vi "DVS_LabVIEW Controller.vi"() -> ()   [LabVIEW 2013]
doc: "This example demonstrates temperature control and monitoring.\n\nNote:\nBefore start this VI is it necessary:\n\n- preconfigure some specific parameters that are not supported by this driver (e.g. PV-I/O Type, Linearization type, Alarm Input Values... ) by Quick Codes, or by Eurotherm iTools or by instrument front panel controls\n- enter correct VISA Resource Descriptor, Device Address and Baud Rate into front-panel controls"
uses:
  <vilib>/Instr/_visa.llb/VISA Event Mechanism.ctl
  <vilib>/Instr/_visa.llb/Select Event Type.ctl
  <vilib>/Utility/file.llb/Write To Spreadsheet File (string).vi
  <vilib>/Instr/_visa.llb/VISA Configure Serial Port (Instr).vi
  <instrlib>/Keithley 24XX/Public/Data/Read (Single Point).vi
  <instrlib>/Keithley 24XX/Keithley 24XX.lvlib
panel:
  in  "stop":bool
  in  "Tab Control":T1(tab)
  in  "Add comments to the data file here and click anywhere outside\nthe comment box to save. The time at which the comment is\nsaved is recorded in the data file.":string
  in  "O2 PUMP":bool
  in  "QCM":bool
  out "Program Errors":errorcluster
  out "Starting Date/Time":string
  in  "Keithley 4200":bool
  in  "Keithley 2420":bool
  in  "J-KEM":bool
  in  "Automatically stop\nmeasurement?":bool
  in  "Stop after elapsed minutes":dbl
  out "Time Elapsed (min)":dbl caption="Elapsed Time (s)"
  in  "RapidOX":bool
  out "Frequency (Hz)":dbl format="%.6e"
  out "Resistance (Ohm)":dbl format="%.6e"
  out "Waveform Chart 7":T2(graph)
  out "Waveform Chart 5":cluster{dbl, dbl}(graph)
  out "Current Temp (C)":dbl
  in  "Temp Setpoint (C)":dbl=25.0
  out "Current Setpoint (C)":dbl
  out "Waveform Chart":cluster{dbl}(graph)
  out "Torr":dbl
  out "%":dbl
  out "atm":dbl
  in  "Com Port":i32(ring) items=["Com 1", "Com 2", "Com 3", "Com 4", "Com 5", "Com 6", "COM 7", "COM 8", "COM 9", "COM 10", "COM 11", "COM 12", "com 13", "COM 14"]
  in  "Baud Rate 2":i32(ring)=2 items=["2400", "4800", "9600", "19200", "38400", "57600", "115200"]
  in  "Com Port 2":i32(ring) items=["Com 1", "Com 2", "Com 3", "Com 4", "Com 5", "Com 6", "COM 7", "COM 8", "COM 9", "COM 10", "COM 11", "COM 12", "com 13", "COM 14"]
  out "Waveform Chart 6":cluster{dbl}(graph)
  out "O2 Concentration (PPM)":dbl
  out "Waveform Chart 4":cluster{"Resistance":sgl}(graph)
  out "Resistance (Ohm)":sgl
  in  "Measurement":enum16{"Resistor/Diode", "Transistor"}(ring)
  out "Waveform Chart 3":cluster{dbl}(graph)
  out "XY Graph":cluster{dbl[], dbl[]}(graph)
  out "Current (A)    Voltage (V)":dbl[][](array[numeric]) caption="appended array"
  out "Resistance (Ohm)":dbl
  # "Configuring Instrument\n \nPlease Wait......\n\nChart will update in 20 sec"
  # "Instruments Connected"
  # "COMMENT BOX"
  # "Instructions:\nSelect the instruments above which are connected, turned on, and configured to record data.\nRun the Pirani Control software, and make sure Pirani is saving a log of the temp/pressure/gas flow data. \nClick the RUN arrow on the LabVIEW toolbar, and wait for instruments to begin recording.\nTo end, click the red STOP button ONLY for instruments that are running.\nDO NOT press the STOP button on the toolbar."
  # "O2 Partial\nPressure"
  # "4-Point Resistance Measurement:\nSMU1 = Current Source, Voltmeter\nSMU2 = COM & GND"
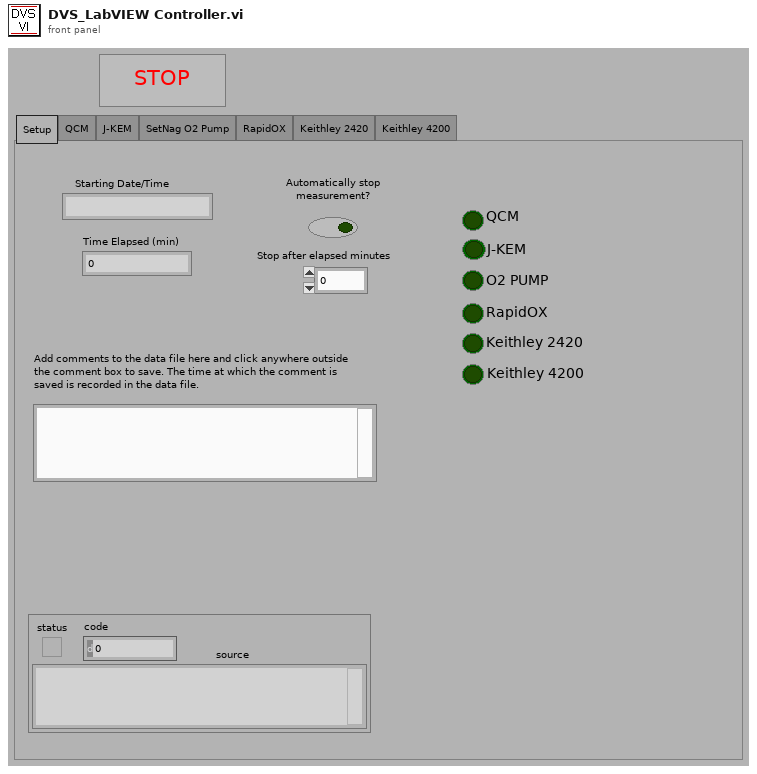
[diagram p1: front panel]
types:
  T1 = enum32{"Setup", "QCM", "J-KEM", "SetNag O2 Pump", "RapidOX", "Keithley 2420", "Keithley 4200"}
  T2 = cluster{"Frequency out":dbl, "Resistance out":dbl}
  T3 = enum16{"open", "open or create", "create or replace", "create", "open (read only)"}
  T4 = enum16{"no parity", "odd parity", "even parity", "mark parity", "space parity"}
  T5 = typedef "Select Event Type.ctl" = u32
  T6 = typedef "VISA Event Mechanism.ctl" = u16
  T7 = cluster{bool, "VISA resource name":refnum<visa-resource-name>, "error out":errorcluster}
  T8 = cluster{bool, "VISA resource name out":refnum<visa-resource-name>, "error out":errorcluster}
  T9 = cluster{bool, "VISA out":refnum<visa-resource-name>, "error out":errorcluster}
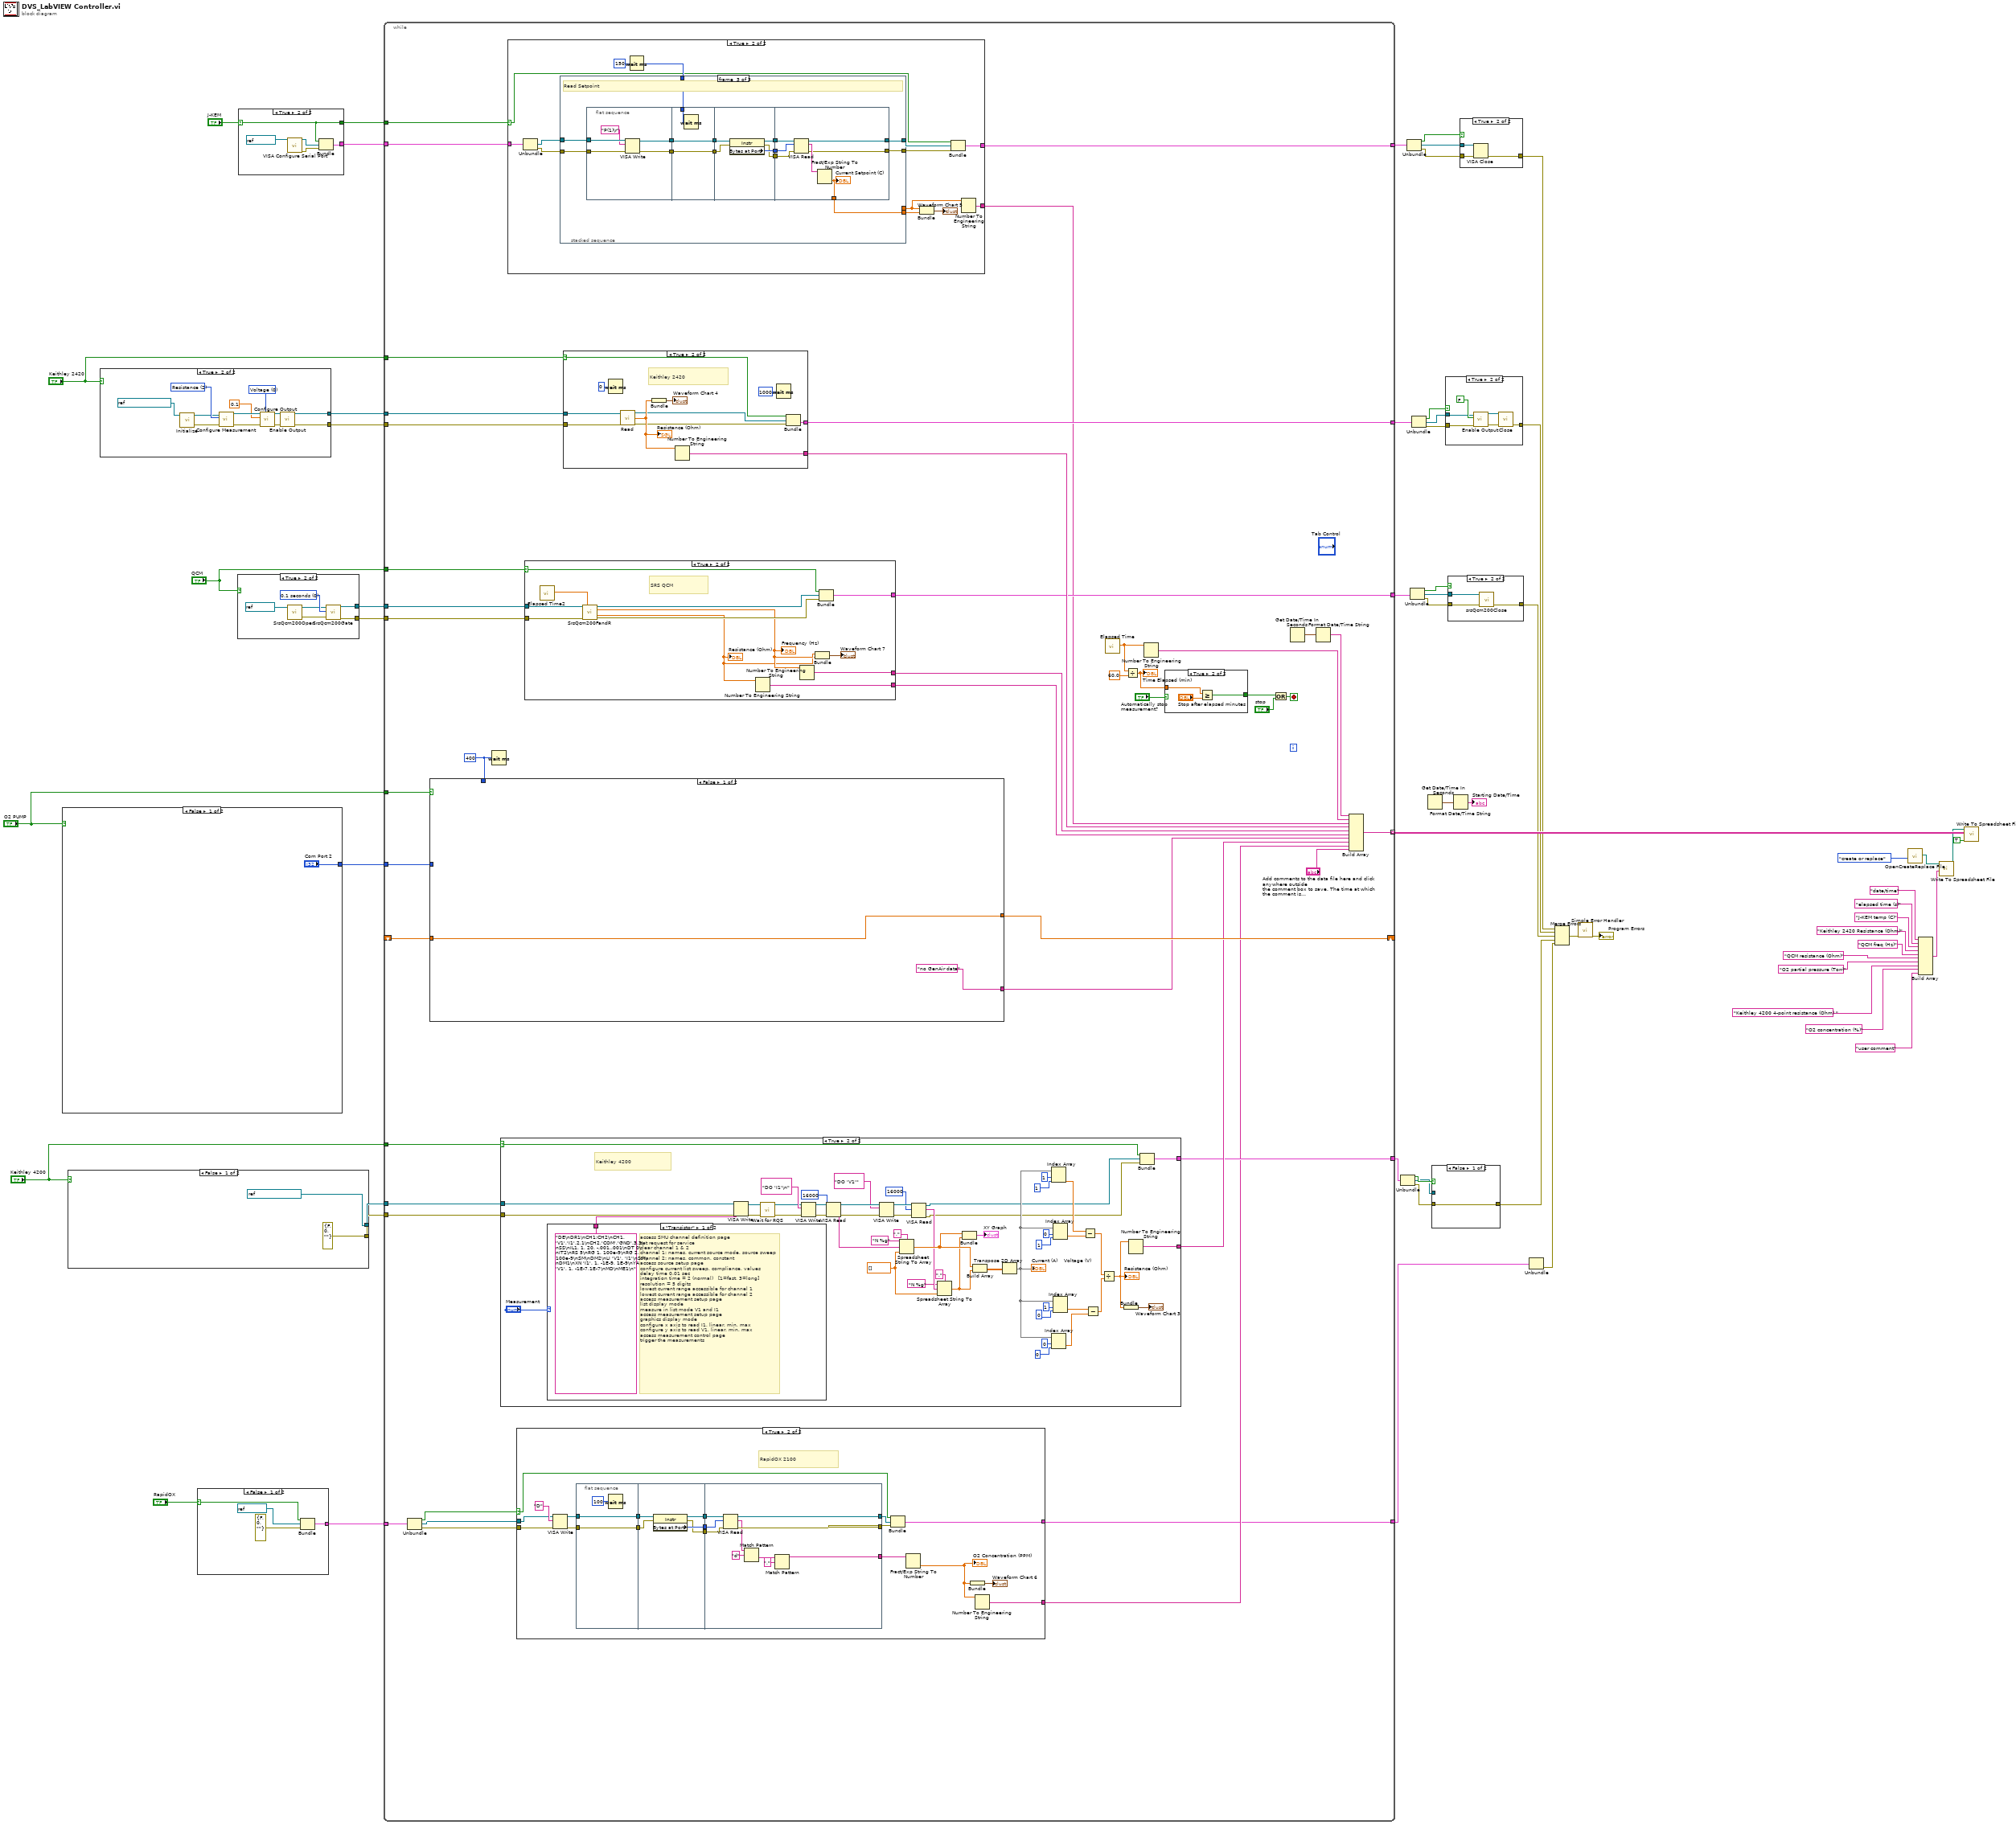
[diagram p0: block diagram]
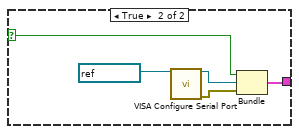
[diagram p2: hidden frame]
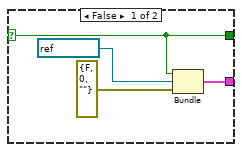
[diagram p4: hidden frame]
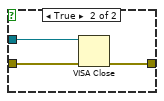
[diagram p5: hidden frame]
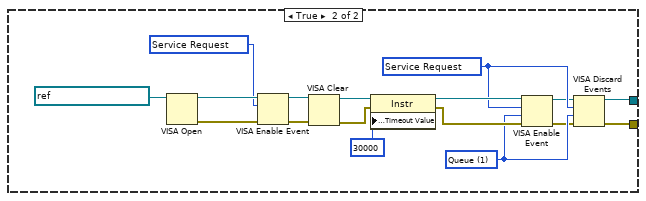
[diagram p6: hidden frame]
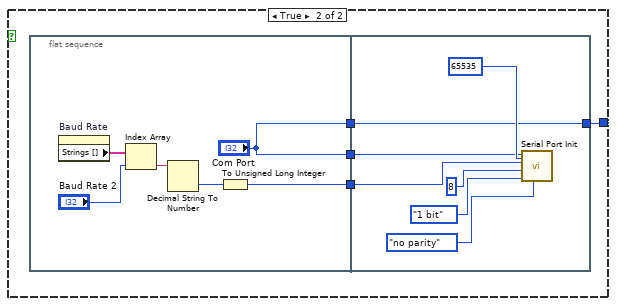
[diagram p7: hidden frame]
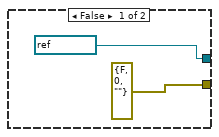
[diagram p9: hidden frame]
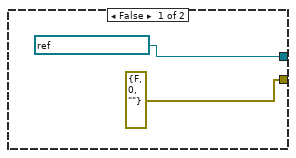
[diagram p11: hidden frame]
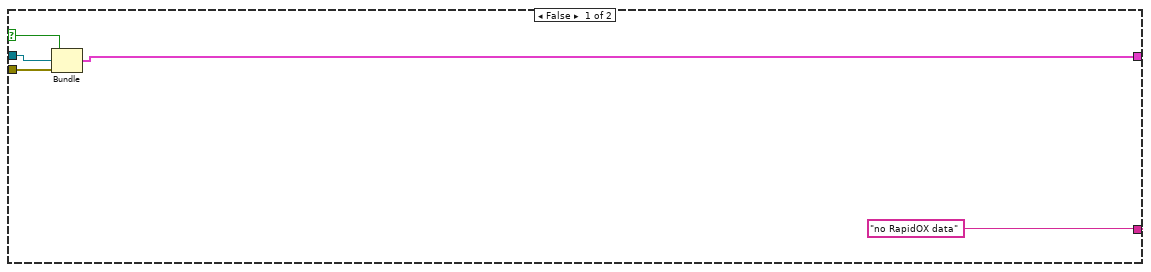
[diagram p12: hidden frame]
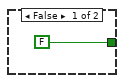
[diagram p13: hidden frame]
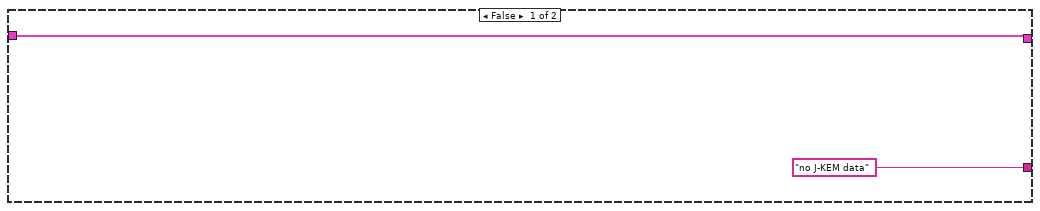
[diagram p14: hidden frame]
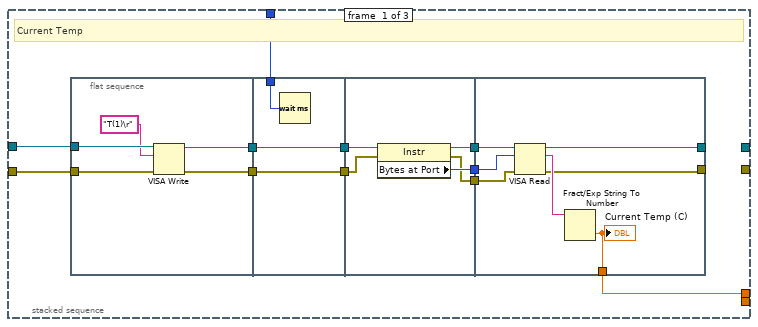
[diagram p15: hidden frame]
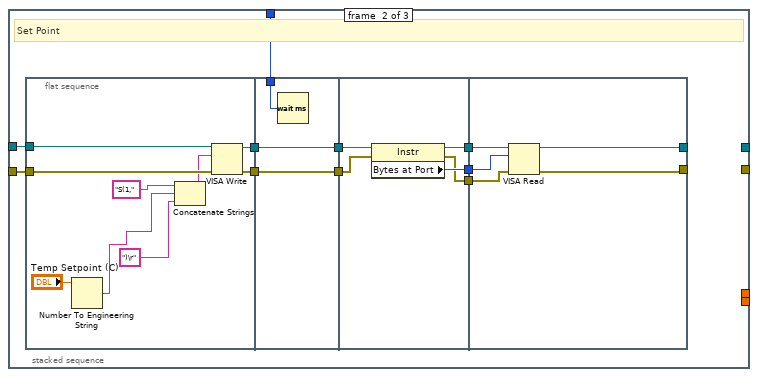
[diagram p16: hidden frame]
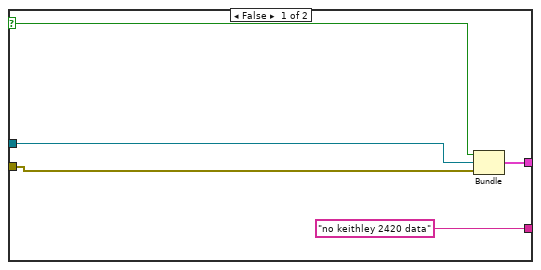
[diagram p17: hidden frame]
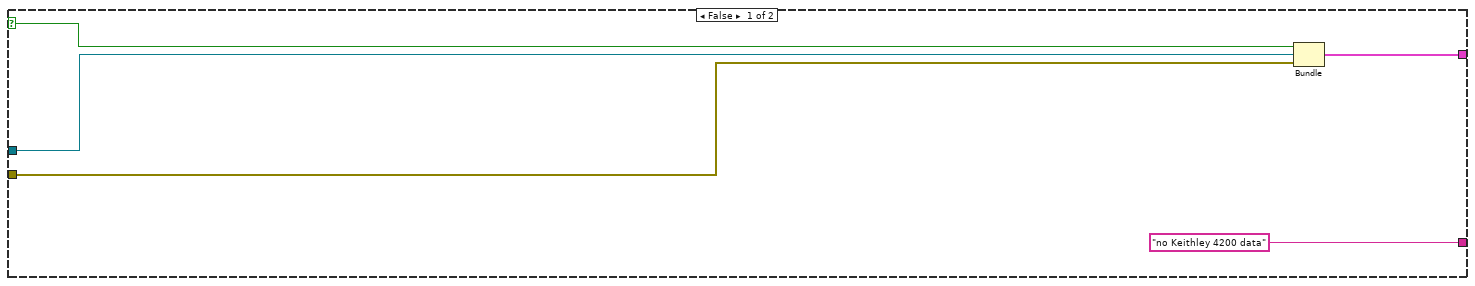
[diagram p18: hidden frame]
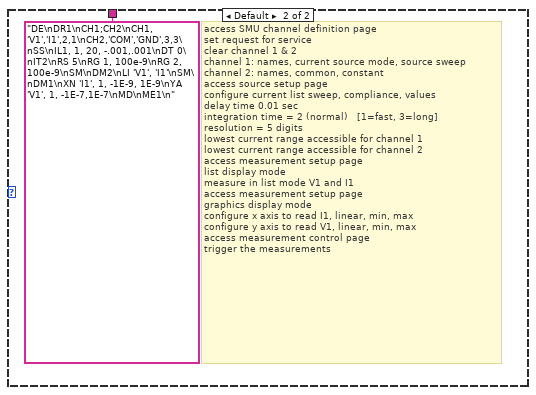
[diagram p19: hidden frame]
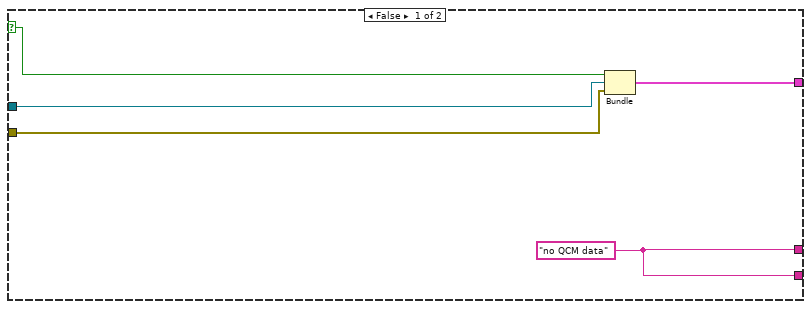
[diagram p20: hidden frame]
diagram:
  n1 = case shown="False" "O2 PUMP" {
    tunnel: ["Com Port 2" w60] -> w46
    frame False {
    }
    frame True {
      n2 = flat-sequence {
        tunnel: ["Com Port"] -> w63
        tunnel: [w65] -> w62
        tunnel: ["Com Port"] -> w61
        tunnel: w63 -> [w71]
        tunnel: w62 -> [w70]
        tunnel: w61 -> [w72]
        tunnel: [w72] -> w60
        frame #0 {
          n3 = property on="Baud Rate" class="Ring (strict)"() -> ("Strings []"=w67:string[])  [unwired: 2 in, 2 out]
          n4 = Index Array(array=w67, index="Baud Rate 2") -> (element=w68:string)
          n5 = Decimal String To Number(string=w68) -> (number=w66:i32)  [unwired: 2 in, 1 out]
          n6 = To Unsigned Long Integer(number=w66) -> (unsigned 32bit integer=w65:u32)
        }
        frame #1 {
          n7 = call <vilib>:"Serial Port Init.vi"("parity"=T4."no parity", "buffer size"=u16 65535, "stop bits"=enum16{"1 bit", "1.5 bits", "2 bits"}."1 bit", "data bits"=u16 8, "baud rate"=w70, "port number"=w71) -> ()  [unwired: 1 in, 1 out]
        }
      }
    }
  }
  n8 = case shown="False" "Keithley 4200" {
    tunnel: [refnum<visa-resource-name> "GPIB0::17::INSTR" ("VISA resource name") w80] -> w42
    tunnel: [errorcluster {"status"=FALSE, "code"=0, "source"=""} ("error out") w79] -> w41
    frame False {
    }
    frame True {
      w92 = T5 1073684491 items=["Service Request"=1073684491, "Trigger"=3221168138, "Clear"=1073684493, "VXI Signal"=1073684512, "VXI/VME Interrupt"=3221168161, "VXI/VME Sysfail"=1073684509, "VXI/VME Sysreset"=1073684510, "GPIB CIC"=1073684498, "GPIB Talk"=1073684499, "GPIB Listen"=1073684500, "PXI Interrupt"=1073684514, "Serial Break"=1073684515, "Serial TermChar"=1073684516, "Serial CTS"=1073684521, "Serial DSR"=1073684522, "Serial DCD"=1073684524, "Serial RI"=1073684526, "Serial Character"=1073684533, "USB Interrupt"=1073684535, "All Enabled"=1073709055] ("Event Type")
      w85 = T6 1 items=["Queue"=1] ("Mechanism Type")
      w84 = T5 1073684491 items=["Service Request"=1073684491, "Trigger"=3221168138, "Clear"=1073684493, "VXI Signal"=1073684512, "VXI/VME Interrupt"=3221168161, "VXI/VME Sysfail"=1073684509, "VXI/VME Sysreset"=1073684510, "GPIB CIC"=1073684498, "GPIB Talk"=1073684499, "GPIB Listen"=1073684500, "PXI Interrupt"=1073684514, "Serial Break"=1073684515, "Serial TermChar"=1073684516, "Serial CTS"=1073684521, "Serial DSR"=1073684522, "Serial DCD"=1073684524, "Serial RI"=1073684526, "Serial Character"=1073684533, "USB Interrupt"=1073684535, "All Enabled"=1073709055] ("Event Type")
      n9 = VISA Open(VISA resource name=refnum<visa-resource-name> "GPIB0::17::INSTR") -> (VISA resource name=w94:refnum<visa-resource-name>, error out=w95:errorcluster)  [unwired: 1 in, 3 out]
      n10 = VISA Enable Event(8:w95, 10:w92, 11:w94) -> (0:w91:errorcluster, 3:w90:refnum<visa-resource-name>)  [unwired: 1 out]
      n11 = VISA Clear(VISA resource name=w90, error in (no error)=w91) -> (VISA resource name out=w86:refnum<visa-resource-name>, error out=w87:errorcluster)
      n12 = property class="Instr"(reference=w86, error in=w87, "General Settings:Timeout Value"=u32 30000) -> (reference out=w88:refnum<visa-resource-name>, error out=w89:errorcluster)
      n13 = VISA Enable Event(8:w89, 9:w85, 10:w84, 11:w88) -> (0:w83:errorcluster, 3:w82:refnum<visa-resource-name>)
      n14 = VISA Discard Events(8:w83, 9:w85, 10:w84, 11:w82) -> (0:w79:errorcluster, 3:w80:refnum<visa-resource-name>)
    }
  }
  n15 = case shown="True" "Keithley 2420" {
    tunnel: [refnum<visa-resource-name> "GPIB1::24::INSTR" ("VISA resource name") w99] -> w52
    tunnel: [errorcluster {"status"=FALSE, "code"=0, "source"=""} ("error out") w98] -> w51
    frame False {
    }
    frame True {
      w103 = u16 0 items=["Voltage", "Current"] ("Source Mode  (0: Voltage)")
      w108 = u16 2 items=["Volts", "Current", "Resistance"] ("Function (0: Volts)")
      n16 = call <instrlib>:"Initialize.vi"("VISA resource name"=refnum<visa-resource-name> "GPIB1::24::INSTR") -> ("error out"=w100:errorcluster, "VISA resource name out"=w101:refnum<visa-resource-name>)  [unwired: 9 in]
      n17 = call <instrlib>:"Configure Measurement.vi"("error in (no error)"=w100, "Function (0: Volts)"=w108, "VISA resource name"=w101) -> ("error out"=w107:errorcluster, "VISA resource name out"=w106:refnum<visa-resource-name>)  [unwired: 7 in]
      n18 = call <instrlib>:"Configure Output.vi"("Source Mode  (0: Voltage)"=w103, "error in (no error)"=w107, "Output Level (0)"=0.1, "VISA resource name"=w106) -> ("error out"=w105:errorcluster, "VISA resource name out"=w104:refnum<visa-resource-name>)  [unwired: 6 in]
      n19 = call <instrlib>:"Enable Output.vi"("error in (no error)"=w105, "VISA resource name"=w104) -> ("error out"=w98:errorcluster, "VISA resource name out"=w99:refnum<visa-resource-name>)  [unwired: 8 in]
    }
  }
  n20 = case shown="False" "RapidOX" {
    selector: "RapidOX" -> [w110 w114]
    tunnel: [w111 w115] -> w4
    frame False {
      n21 = Bundle(w110, "VISA resource name"=refnum<visa-resource-name> "COM7", "error out"=errorcluster {"status"=FALSE, "code"=0, "source"=""}) -> (w111:T7)  [unwired: 1 in]
    }
    frame True {
      n22 = call-poly "VISA Configure Serial Port"("VISA resource name"=refnum<visa-resource-name> "COM7") -> ("VISA resource name out"=w117:refnum<visa-resource-name>, "error out"=w116:errorcluster)  [unwired: 13 in]
      n23 = Bundle(w114, "VISA resource name out"=w117, "error out"=w116) -> (w115:T8)  [unwired: 1 in]
    }
  }
  n24 = case shown="True" "QCM" {
    tunnel: [refnum<visa-resource-name> "COM6" ("VISA in") w122] -> w50
    tunnel: [errorcluster {"status"=FALSE, "code"=0, "source"=""} ("error out") w121] -> w49
    frame False {
    }
    frame True {
      w126 = u16 0 items=["0.1 seconds", "1.0 seconds", "10.0 seconds"] ("Gate in")
      n25 = call <instrlib>:"SrsQcm200Open.vi"("VISA in"=refnum<visa-resource-name> "COM6") -> ("error out"=w123:errorcluster, "VISA out"=w124:refnum<visa-resource-name>)  [unwired: 4 in]
      n26 = call <instrlib>:"SrsQcm200Gate.vi"("VISA in"=w124, "Gate in"=w126, "error in (no error)"=w123) -> ("VISA out"=w122:refnum<visa-resource-name>, "error out"=w121:errorcluster)  [unwired: 14 in, 1 out]
    }
  }
  n27 = case shown="True" "J-KEM" {
    selector: "J-KEM" -> [w127 w131]
    tunnel: [w128 w132] -> w28
    tunnel: [w127 w131] -> w20
    frame False {
      n28 = Bundle(w127, "VISA resource name"=refnum<visa-resource-name> "COM3", "error out"=errorcluster {"status"=FALSE, "code"=0, "source"=""}) -> (w128:T7)  [unwired: 1 in]
    }
    frame True {
      n29 = call-poly "VISA Configure Serial Port"("VISA resource name"=refnum<visa-resource-name> "COM3") -> ("VISA resource name out"=w134:refnum<visa-resource-name>, "error out"=w133:errorcluster)  [unwired: 13 in]
      n30 = Bundle(w131, "VISA resource name out"=w134, "error out"=w133) -> (w132:T8)  [unwired: 1 in]
    }
  }
  n31 = while {
    shift-right: [w177] -> _
    shift-left: _ -> [w176]
    tunnel: [w173] -> w54 mode=indexing
    tunnel: "Keithley 2420" -> [w169]
    tunnel: w52 -> [w171]
    tunnel: w51 -> [w170]
    tunnel: w50 -> [w168]
    tunnel: w49 -> [w167]
    tunnel: "QCM" -> [w165]
    tunnel: "O2 PUMP" -> [w154]
    tunnel: w46 -> [w164]
    tunnel: "Keithley 4200" -> [w158]
    tunnel: w42 -> [w163]
    tunnel: w41 -> [w162]
    tunnel: [w156] -> w40
    tunnel: [w155] -> w36
    tunnel: [w153] -> w32
    tunnel: w28 -> [w152]
    tunnel: [w151] -> w26
    tunnel: w20 -> [w149]
    tunnel: w4 -> [w141]
    tunnel: [w136] -> w2
    stop <- w147 stop-if-true
    w175 = u32 400 ("milliseconds to wait")
    n32 = Unbundle(w141) -> (w140:bool, "VISA resource name out"=w139:refnum<visa-resource-name>, "error out"=w138:errorcluster)
    n33 = case shown="False" w154 {
      tunnel: [w427 w431] -> w177
      tunnel: w176 -> [w427 w432]
      tunnel: w175 -> [_ w428]
      tunnel: w164 -> [_ w430]
      tunnel: ["no GenAir data" w429] -> w161
      frame False {
      }
      frame True {
        # "SetNag O2 Gauge"
        n34 = flat-sequence {
          tunnel: [w441] -> w438
          tunnel: w428 -> [w443]
          tunnel: w430 -> [w441]
          tunnel: w438 -> [w444]
          tunnel: w428 -> [w451]
          tunnel: [w447] -> w431
          frame #0 {
            n35 = Wait (ms)(milliseconds to wait=w443) -> ()  [unwired: 1 out]
            n36 = call <vilib>:"Serial Port Write.vi"("string to write"="_OXY\r" ("O2 partial press"), "port number"=w441) -> ()  [unwired: 1 out]
          }
          frame #1 {
            # "O2 partial pressure"
            n37 = call <vilib>:"Bytes At Serial Port.vi"() -> ("byte count"=w452:u32)  [unwired: 1 in, 1 out]
            n38 = Wait (ms)(milliseconds to wait=w451) -> ()  [unwired: 1 out]
            n39 = call <vilib>:"Serial Port Read.vi"("requested byte count"=w452, "port number"=w444) -> ("string read"=w450:string)  [unwired: 1 out]
            n40 = Fract/Exp String To Number(string=w450) -> (number=w448:dbl)  [unwired: 3 in, 1 out]
            "atm" <- w448
            n41 = Multiply(x=w448, y=100.0) -> (x*y=w445:dbl)
            "%" <- w445
            n42 = Multiply(x=w445, y=7.6) -> (x*y=w447:dbl)
            "Torr" <- w447
          }
        }
        n43 = Wait (ms)(milliseconds to wait=w428) -> ()  [unwired: 1 out]
        n44 = Greater?(x=w431, y=1e-07) -> (0:w434:bool)
        n45 = case shown="False" w434 {
          tunnel: [w439 w440] -> w433
          tunnel: w431 -> [_ w440]
          tunnel: w432 -> [w439 _]
          frame False {
          }
          frame True {
          }
        }
        n46 = Number To Engineering String(4:w433) -> (0:w429:string)  [unwired: 3 in]
        n47 = Bundle(w429) -> (w436:cluster{string})  [unwired: 1 in]
        n48 = Fract/Exp String To Number(string=w436) -> (number=→"Waveform Chart":cluster{dbl})  [unwired: 3 in, 1 out]
      }
    }
    n49 = Wait (ms)(milliseconds to wait=w175) -> ()  [unwired: 1 out]
    n50 = case shown="True" w158 {
      selector: w158 -> [w352 w358]
      tunnel: w163 -> [w354 w363]
      tunnel: w162 -> [w353 w362]
      tunnel: ["no Keithley 4200 data" w361] -> w159
      tunnel: [w351 w357] -> w153
      frame False {
        n51 = Bundle(w352, "VISA resource name"=w354, "error out"=w353) -> (w351:T7)  [unwired: 1 in]
      }
      frame True {
        w396 = dbl[] []
        # "Keithley 4200"
        n52 = case shown="\"Transistor\"" "Measurement" {
          tunnel: ["DE\nDR1\nCH1;CH2\nCH1, 'V1','I1',2,1\nCH2,'COM','GND',3,3\nSS\nIL1, 1, 20, -.001,.001\nDT 0\nIT2\nRS 5\nRG 1, 100e-9\nRG 2, 100e-9\nSM\nDM2\nLI 'V1', 'I1'\nSM\nDM1\nXN 'I1', 1, -1E-9, 1E-9\nYA 'V1', 1, -1E-7,1E-7\nMD\nME1\n" ("write buffer") "DE\nDR1\nCH1;CH2\nCH1, 'V1','I1',2,1\nCH2,'COM','GND',3,3\nSS\nIL1, 1, 20, -.001,.001\nDT 0\nIT2\nRS 5\nRG 1, 100e-9\nRG 2, 100e-9\nSM\nDM2\nLI 'V1', 'I1'\nSM\nDM1\nXN 'I1', 1, -1E-9, 1E-9\nYA 'V1', 1, -1E-7,1E-7\nMD\nME1\n" ("write buffer")] -> w370
          frame "Transistor" {
            # "access SMU channel definition page\nset request for service\nclear channel 1 & 2\nchannel 1: names, current source mode, source sweep\nchannel 2: names, common, constant\naccess source setup page\nconfigure current list sweep, compliance, values\ndelay time 0.01 sec\nintegration time = 2 (normal)   [1=fast, 3=long]\nresolution = 5 digits\nlowest current range accessible for channel 1\nlowest current range accessible for channel 2\naccess measurement setup page\nlist display mode\nmeasure in list mode V1 and I1\naccess measurement setup page\ngraphics display mode\nconfigure x axis to read I1, linear, min, max\nconfigure y axis to read V1, linear, min, max\naccess measurement control page\ntrigger the measurements"
          }
          frame Default {
            # "access SMU channel definition page\nset request for service\nclear channel 1 & 2\nchannel 1: names, current source mode, source sweep\nchannel 2: names, common, constant\naccess source setup page\nconfigure current list sweep, compliance, values\ndelay time 0.01 sec\nintegration time = 2 (normal)   [1=fast, 3=long]\nresolution = 5 digits\nlowest current range accessible for channel 1\nlowest current range accessible for channel 2\naccess measurement setup page\nlist display mode\nmeasure in list mode V1 and I1\naccess measurement setup page\ngraphics display mode\nconfigure x axis to read I1, linear, min, max\nconfigure y axis to read V1, linear, min, max\naccess measurement control page\ntrigger the measurements"
          }
        }
        n53 = VISA Write(VISA resource name=w363, write buffer=w370, error in (no error)=w362) -> (VISA resource name out=w371:refnum<visa-resource-name>, error out=w372:errorcluster)  [unwired: 1 out]
        n54 = call <vilib>:"Wait for RQS.vi"("error in (no error)"=w372, "VISA resource name"=w371) -> ("error out"=w368:errorcluster, "VISA resource name out"=w369:refnum<visa-resource-name>)  [unwired: 1 in, 7 out]
        n55 = VISA Write(VISA resource name=w369, write buffer="DO 'I1'\n", error in (no error)=w368) -> (VISA resource name out=w406:refnum<visa-resource-name>, error out=w402:errorcluster)  [unwired: 1 out]
        n56 = VISA Read(VISA resource name=w406, byte count=u32 16000, error in (no error)=w402) -> (VISA resource name out=w404:refnum<visa-resource-name>, read buffer=w389:string, error out=w400:errorcluster)  [unwired: 1 out]
        n57 = VISA Write(VISA resource name=w404, write buffer="DO 'V1'", error in (no error)=w400) -> (VISA resource name out=w398:refnum<visa-resource-name>, error out=w399:errorcluster)  [unwired: 1 out]
        n58 = Spreadsheet String To Array(delimiter (Tab)=",", format string="N %g", spreadsheet string=w389, array type (2D Dbl)=w396) -> (array=w393:dbl[])
        n59 = VISA Read(VISA resource name=w398, byte count=u32 16000, error in (no error)=w399) -> (VISA resource name out=w360:refnum<visa-resource-name>, read buffer=w388:string, error out=w359:errorcluster)  [unwired: 1 out]
        n60 = Spreadsheet String To Array(delimiter (Tab)=",", format string="N %g", spreadsheet string=w388, array type (2D Dbl)=w396) -> (array=w392:dbl[])
        n61 = Bundle(w393, w392) -> (→"XY Graph":cluster{dbl[], dbl[]})  [unwired: 1 in]
        n62 = Build Array(w393, w392) -> (w390:dbl[][])
        n63 = Transpose 2D Array(2D array=w390) -> (transposed array=w375:dbl[][])
        "Current (A)    Voltage (V)" <- w375
        n64 = Index Array(array=w375, index (row)=1, index (col)=1 ("index (row)")) -> (element=w377:dbl)
        n65 = Index Array(array=w375, index (row)=0, index (col)=0 ("index (row)")) -> (element=w378:dbl)
        n66 = Index Array(array=w375, index (row)=0, index (col)=1 ("index (row)")) -> (element=w376:dbl)
        n67 = Index Array(array=w375, index (row)=1, index (col)=0 ("index (row)")) -> (element=w379:dbl)
        n68 = Subtract(x=w377, y=w376) -> (x-y=w373:dbl)
        n69 = Subtract(x=w379, y=w378) -> (x-y=w374:dbl)
        n70 = Divide(x=w373, y=w374) -> (x/y=w364:dbl)
        "Resistance (Ohm)" <- w364
        n71 = Bundle(w364) -> (→"Waveform Chart 3":cluster{dbl})  [unwired: 1 in]
        n72 = Number To Engineering String(4:w364) -> (0:w361:string)  [unwired: 3 in]
        n73 = Bundle(w358, "VISA resource name out"=w360, "error out"=w359) -> (w357:T8)  [unwired: 1 in]
      }
    }
    n74 = case shown="True" w149 {
      selector: w149 -> [_ w227]
      tunnel: w152 -> [w226 w233]
      tunnel: [w226 w230] -> w151
      tunnel: ["no J-KEM data" w228] -> w150
      frame False {
      }
      frame True {
        w238 = u32 150 ("milliseconds to wait")
        n75 = Unbundle(w233) -> ("VISA resource name out"=w232:refnum<visa-resource-name>, "error out"=w231:errorcluster)  [unwired: 1 out]
        n76 = stacked-sequence {
          tunnel: w232 -> [w242 w272 w306]
          tunnel: w231 -> [w241 w271 w305]
          tunnel: w238 -> [w240 w270 w307]
          tunnel: [_ _ w304] -> w234
          tunnel: [_ _ w303] -> w235
          tunnel: [w239 _ _] -> w229
          tunnel: [_ _ w302] -> w237
          frame #0 {
            # "Current Temp"
            n77 = flat-sequence {
              tunnel: w242 -> [w254]
              tunnel: w241 -> [w253]
              tunnel: [w251] -> w249
              tunnel: [w250] -> w248
              tunnel: w240 -> [w257]
              tunnel: [w256] -> w247
              tunnel: w249 -> [w256]
              tunnel: w248 -> [w255]
              tunnel: [w255] -> w246
              tunnel: w247 -> [w262]
              tunnel: w246 -> [w261]
              tunnel: [w260] -> w245
              tunnel: [w259] -> w244
              tunnel: [w258] -> w243
              tunnel: w245 -> [w269]
              tunnel: w244 -> [w268]
              tunnel: w243 -> [w267]
              tunnel: [w264] -> _
              tunnel: [w265] -> _
              tunnel: [w263] -> w239
              frame #0 {
                n78 = VISA Write(VISA resource name=w254, write buffer="T(1)\r", error in (no error)=w253) -> (VISA resource name out=w251:refnum<visa-resource-name>, error out=w250:errorcluster)  [unwired: 1 out]
              }
              frame #1 {
                n79 = Wait (ms)(milliseconds to wait=w257) -> ()  [unwired: 1 out]
              }
              frame #2 {
                n80 = property class="Instr"(reference=w262, error in=w261) -> (reference out=w260:refnum<visa-resource-name>, error out=w258:errorcluster, "Bytes at Port"=w259:u32)
              }
              frame #3 {
                n81 = VISA Read(VISA resource name=w269, byte count=w268, error in (no error)=w267) -> (VISA resource name out=w265:refnum<visa-resource-name>, read buffer=w266:string, error out=w264:errorcluster)  [unwired: 1 out]
                n82 = Fract/Exp String To Number(string=w266) -> (number=w263:dbl)  [unwired: 3 in, 1 out]
                "Current Temp (C)" <- w263
              }
            }
          }
          frame #1 {
            # "Set Point"
            n83 = flat-sequence {
              tunnel: w272 -> [w288]
              tunnel: w271 -> [w287]
              tunnel: [w286] -> w279
              tunnel: [w285] -> w278
              tunnel: w270 -> [w291]
              tunnel: [w290] -> w277
              tunnel: w279 -> [w290]
              tunnel: w278 -> [w289]
              tunnel: [w289] -> w276
              tunnel: w277 -> [w296]
              tunnel: w276 -> [w295]
              tunnel: [w294] -> w275
              tunnel: [w293] -> w274
              tunnel: [w292] -> w273
              tunnel: w275 -> [w301]
              tunnel: w274 -> [w300]
              tunnel: w273 -> [w299]
              tunnel: [w297] -> _
              tunnel: [w298] -> _
              frame #0 {
                n84 = Number To Engineering String(4:"Temp Setpoint (C)") -> (0:w281:string)  [unwired: 3 in]
                n85 = Concatenate Strings("S(1," ("write buffer"), w281, ")\r" ("write buffer")) -> (w284:string)
                n86 = VISA Write(VISA resource name=w288, write buffer=w284, error in (no error)=w287) -> (VISA resource name out=w286:refnum<visa-resource-name>, error out=w285:errorcluster)  [unwired: 1 out]
              }
              frame #1 {
                n87 = Wait (ms)(milliseconds to wait=w291) -> ()  [unwired: 1 out]
              }
              frame #2 {
                n88 = property class="Instr"(reference=w296, error in=w295) -> (reference out=w294:refnum<visa-resource-name>, error out=w292:errorcluster, "Bytes at Port"=w293:u32)
              }
              frame #3 {
                n89 = VISA Read(VISA resource name=w301, byte count=w300, error in (no error)=w299) -> (VISA resource name out=w298:refnum<visa-resource-name>, error out=w297:errorcluster)  [unwired: 2 out]
              }
            }
          }
          frame #2 {
            # "Read Setpoint"
            n90 = flat-sequence {
              tunnel: w306 -> [w319]
              tunnel: w305 -> [w318]
              tunnel: [w316] -> w314
              tunnel: [w315] -> w313
              tunnel: [w322] -> w312
              tunnel: w314 -> [w322]
              tunnel: w313 -> [w321]
              tunnel: [w321] -> w311
              tunnel: w307 -> [w320]
              tunnel: w312 -> [w327]
              tunnel: w311 -> [w326]
              tunnel: [w325] -> w310
              tunnel: [w324] -> w309
              tunnel: [w323] -> w308
              tunnel: w310 -> [w334]
              tunnel: w309 -> [w333]
              tunnel: w308 -> [w332]
              tunnel: [w329] -> w303
              tunnel: [w330] -> w304
              tunnel: [w328] -> w302
              frame #0 {
                n91 = VISA Write(VISA resource name=w319, write buffer="P(1)\r", error in (no error)=w318) -> (VISA resource name out=w316:refnum<visa-resource-name>, error out=w315:errorcluster)  [unwired: 1 out]
              }
              frame #1 {
                n92 = Wait (ms)(milliseconds to wait=w320) -> ()  [unwired: 1 out]
              }
              frame #2 {
                n93 = property class="Instr"(reference=w327, error in=w326) -> (reference out=w325:refnum<visa-resource-name>, error out=w323:errorcluster, "Bytes at Port"=w324:u32)
              }
              frame #3 {
                n94 = VISA Read(VISA resource name=w334, byte count=w333, error in (no error)=w332) -> (VISA resource name out=w330:refnum<visa-resource-name>, read buffer=w331:string, error out=w329:errorcluster)  [unwired: 1 out]
                n95 = Fract/Exp String To Number(string=w331) -> (number=w328:dbl)  [unwired: 3 in, 1 out]
                "Current Setpoint (C)" <- w328
              }
            }
          }
        }
        n96 = Wait (ms)(milliseconds to wait=w238) -> ()  [unwired: 1 out]
        n97 = Bundle(w229, w237) -> (→"Waveform Chart 5":cluster{dbl, dbl})  [unwired: 1 in]
        n98 = Bundle(w227, "VISA resource name out"=w234, "error out"=w235) -> (w230:T8)  [unwired: 1 in]
        n99 = Number To Engineering String(4:w229) -> (0:w228:string)  [unwired: 3 in]
      }
    }
    n100 = case shown="True" w140 {
      selector: w140 -> [w182 w191]
      tunnel: w139 -> [w183 w190]
      tunnel: w138 -> [w181 w189]
      tunnel: ["no RapidOX data" w188] -> w137
      tunnel: [w180 w187] -> w136
      frame False {
        n101 = Bundle(w182, "VISA resource name out"=w183, "error out"=w181) -> (w180:T8)  [unwired: 1 in]
      }
      frame True {
        # "RapidOX 2100"
        n102 = VISA Write(VISA resource name=w190, write buffer="D", error in (no error)=w189) -> (VISA resource name out=w194:refnum<visa-resource-name>, error out=w193:errorcluster)  [unwired: 1 out]
        n103 = flat-sequence {
          tunnel: [w205] -> w202
          tunnel: [w204] -> w201
          tunnel: w194 -> [w205]
          tunnel: w193 -> [w204]
          tunnel: w202 -> [w210]
          tunnel: w201 -> [w209]
          tunnel: [w208] -> w200
          tunnel: [w207] -> w199
          tunnel: [w206] -> w198
          tunnel: w200 -> [w220]
          tunnel: w199 -> [w219]
          tunnel: w198 -> [w218]
          tunnel: [w216] -> w196
          tunnel: [w217] -> w197
          tunnel: [w211] -> w186
          frame #0 {
            n104 = Wait (ms)(milliseconds to wait=u32 100) -> ()  [unwired: 1 out]
          }
          frame #1 {
            n105 = property class="Instr"(reference=w210, error in=w209) -> (reference out=w208:refnum<visa-resource-name>, error out=w206:errorcluster, "Bytes at Port"=w207:u32)
          }
          frame #2 {
            n106 = VISA Read(VISA resource name=w220, byte count=w219, error in (no error)=w218) -> (VISA resource name out=w217:refnum<visa-resource-name>, read buffer=w214:string, error out=w216:errorcluster)  [unwired: 1 out]
            n107 = Match Pattern(string=w214, regular expression="d") -> (after substring=w212:string)  [unwired: 1 in, 3 out]
            n108 = Match Pattern(string=w212, regular expression=",") -> (before substring=w211:string)  [unwired: 1 in, 3 out]
          }
        }
        n109 = Bundle(w191, "VISA resource name out"=w197, "error out"=w196) -> (w187:T8)  [unwired: 1 in]
        n110 = Fract/Exp String To Number(string=w186) -> (number=w185:dbl)  [unwired: 3 in, 1 out]
        "O2 Concentration (PPM)" <- w185
        n111 = Bundle(w185) -> (→"Waveform Chart 6":cluster{dbl})  [unwired: 1 in]
        n112 = Number To Engineering String(4:w185) -> (0:w188:string)  [unwired: 3 in]
      }
    }
    n113 = case shown="True" w165 {
      selector: w165 -> [w412 w418]
      tunnel: w168 -> [w411 w424]
      tunnel: w167 -> [w410 w423]
      tunnel: [w413 w422] -> w166
      tunnel: [w413 w421] -> w160
      tunnel: [w409 w417] -> w155
      frame False {
        w413 = "no QCM data"
        n114 = Bundle(w412, "VISA out"=w411, "error out"=w410) -> (w409:T9)  [unwired: 1 in]
      }
      frame True {
        # "SRS QCM"
        n115 = call "Elapsed Time2"() -> ("Elapsed Time (s)"=w425:dbl)  [unwired: 12 in, 7 out]
        n116 = call <instrlib>:"SrsQcm200FandR.vi"("VISA in"=w424, "Reference time in"=w425, "error in (no error)"=w423) -> ("VISA out"=w420:refnum<visa-resource-name>, "Frequency out"=w415:dbl, "Resistance out"=w414:dbl, "error out"=w419:errorcluster)  [unwired: 6 in, 3 out]
        "Frequency (Hz)" <- w415
        "Resistance (Ohm)" <- w414
        n117 = Number To Engineering String(4:w414) -> (0:w421:string)  [unwired: 3 in]
        n118 = Number To Engineering String(4:w415) -> (0:w422:string)  [unwired: 3 in]
        n119 = Bundle("Frequency out"=w415, "Resistance out"=w414) -> (→"Waveform Chart 7":T2)  [unwired: 1 in]
        n120 = Bundle(w418, "VISA out"=w420, "error out"=w419) -> (w417:T9)  [unwired: 1 in]
      }
    }
    n121 = case shown="True" w169 {
      selector: w169 -> [w338 w344]
      tunnel: w171 -> [w337 w346]
      tunnel: w170 -> [w336 w347]
      tunnel: [w335 w342] -> w156
      tunnel: ["no keithley 2420 data" w341] -> w157
      frame False {
        n122 = Bundle(w338, "VISA resource name out"=w337, "error out"=w336) -> (w335:T8)  [unwired: 1 in]
      }
      frame True {
        # "Keithley 2420"
        n123 = Wait (ms)(milliseconds to wait=u32 0) -> ()  [unwired: 1 out]
        n124 = call-poly <instrlib>:"Read.vi"("VISA resource name"=w346, "error in (no error)"=w347) -> ("VISA resource name out"=w345:refnum<visa-resource-name>, "Resistance"=w349:sgl, "error out"=w343:errorcluster)  [unwired: 7 in, 4 out]
        "Resistance (Ohm)" <- w349
        n125 = Bundle("Resistance"=w349) -> (→"Waveform Chart 4":cluster{"Resistance":sgl})  [unwired: 1 in]
        n126 = Number To Engineering String(4:w349) -> (0:w341:string)  [unwired: 3 in]
        n127 = Wait (ms)(milliseconds to wait=u32 1000) -> ()  [unwired: 1 out]
        n128 = Bundle(w344, "VISA resource name out"=w345, "error out"=w343) -> (w342:T8)  [unwired: 1 in]
      }
    }
    n129 = call "Elapsed Time"() -> ("Elapsed Time (s)"=w146:dbl)  [unwired: 12 in, 7 out]
    n130 = Divide(x=w146, y=60.0) -> (x/y=w144:dbl)
    "Time Elapsed (min)" <- w144
    n131 = Number To Engineering String(4:w146) -> (0:w178:string)  [unwired: 3 in]
    n132 = case shown="True" "Automatically stop\nmeasurement?" {
      tunnel: w144 -> [_ w223]
      tunnel: [FALSE w222] -> w142
      frame False {
      }
      frame True {
        n133 = Greater Or Equal?(x=w223, y="Stop after elapsed minutes") -> (x >= y?=w222:bool)
      }
    }
    n134 = Or(x=w142, y="stop") -> (x .or. y?=w147:bool)
    n135 = Get Date/Time In Seconds() -> (seconds since 1Jan1904=w179:timestamp)
    n136 = Format Date/Time String(seconds (now)=w179) -> (date/time string=w172:string)  [unwired: 2 in]
    n137 = Build Array(w172, w178, w150, w157, w166, w160, w161, w159, w137, "Add comments to the data file here and click anywhere outside\nthe comment box to save. The time at which the comment is\nsaved is recorded in the data file.") -> (w173:string[])
  }
  n138 = Unbundle(w32) -> (w31:bool, "VISA resource name out"=w30:refnum<visa-resource-name>, "error out"=w29:errorcluster)
  n139 = Unbundle(w26) -> (w25:bool, "VISA resource name out"=w24:refnum<visa-resource-name>, "error out"=w23:errorcluster)
  n140 = Unbundle(w36) -> (w35:bool, "VISA out"=w34:refnum<visa-resource-name>, "error out"=w33:errorcluster)
  n141 = Unbundle(w40) -> (w39:bool, "VISA resource name out"=w38:refnum<visa-resource-name>, "error out"=w37:errorcluster)
  n142 = Get Date/Time In Seconds() -> (seconds since 1Jan1904=w57:timestamp)
  n143 = case shown="False" w31 {
    tunnel: w30 -> [_ w456]
    tunnel: w29 -> [w453 w455]
    tunnel: [w453 w454] -> w21
    frame False {
    }
    frame True {
      n144 = VISA Close(VISA resource name=w456, error in (no error)=w455) -> (error out=w454:errorcluster)
    }
  }
  n145 = case shown="True" w39 {
    tunnel: w38 -> [_ w460]
    tunnel: w37 -> [w457 w459]
    tunnel: [w457 w458] -> w44
    frame False {
    }
    frame True {
      n146 = call <instrlib>:"Enable Output.vi"("error in (no error)"=w459, "Enable Output (T: Enable)"=FALSE, "VISA resource name"=w460) -> ("error out"=w461:errorcluster, "VISA resource name out"=w463:refnum<visa-resource-name>)  [unwired: 7 in]
      n147 = call <instrlib>:"Close.vi"("error in (no error)"=w461, "VISA resource name"=w463) -> ("error out"=w458:errorcluster)  [unwired: 9 in]
    }
  }
  n148 = case shown="True" w35 {
    tunnel: w33 -> [w464 w467]
    tunnel: [w464 w466] -> w45
    tunnel: w34 -> [_ w465]
    frame False {
    }
    frame True {
      n149 = call <instrlib>:"srsQcm200Close.vi"("error in"=w467, "Visa in"=w465) -> ("error out"=w466:errorcluster)  [unwired: 3 in]
    }
  }
  n150 = Format Date/Time String(seconds (now)=w57) -> (date/time string=→"Starting Date/Time":string)  [unwired: 2 in]
  n151 = case shown="True" w25 {
    tunnel: w24 -> [_ w471]
    tunnel: w23 -> [w468 w470]
    tunnel: [w468 w469] -> w22
    frame False {
    }
    frame True {
      n152 = VISA Close(VISA resource name=w471, error in (no error)=w470) -> (error out=w469:errorcluster)
    }
  }
  n153 = Unbundle(w2) -> ("error out"=w1:errorcluster)  [unwired: 2 out]
  n154 = Merge Errors(w22, w44, w45, w21, w1) -> (w55:errorcluster)
  n155 = call <vilib>:"Simple Error Handler.vi"("error in (no error)"=w55) -> ("error out"=→"Program Errors":errorcluster)  [unwired: 4 in, 4 out]
  n156 = call <instrlib>:"OpenCreateReplace File.vi"("function (open:0)"=T3."create or replace") -> ("new file path"=w9:path)  [unwired: 7 in, 3 out]
  n157 = Build Array("date/time", "elapsed time (s)", "J-KEM temp (C)", "Keithley 2420 Resistance (Ohm)" ("element"), "QCM freq (Hz)", "QCM resistance (Ohm)", "O2 partial pressure (Torr)" ("element"), "Keithley 4200 4-point resistance (Ohm) " ("element"), "O2 concentration (%)" ("element"), "user comment" ("element")) -> (w12:string[])
  n158 = call-poly <vilib>:"Write To Spreadsheet File.vi"("1D data"=w12, "file path (dialog if empty)"=w9) -> ("new file path (Not A Path if cancelled)"=w13:path)  [unwired: 6 in]
  n159 = call-poly <vilib>:"Write To Spreadsheet File.vi"("append to file? (new file:F)"=TRUE, "2D data"=w54, "file path (dialog if empty)"=w13) -> ()  [unwired: 5 in, 1 out]
